vi "Get System Name.vi"() -> (3 "System Name":string)   [LabVIEW 2016]
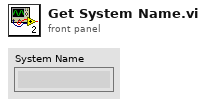
[diagram p1: front panel]
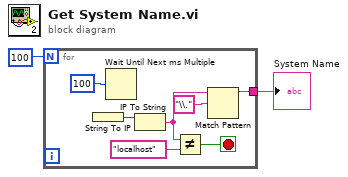
[diagram p0: block diagram]
diagram:
  n1 = for {
    N: 100 -> [_]
    tunnel: [w8] -> w2
    stop <- w5 stop-if-true
    n2 = String To IP() -> (0:w7:u32)  [unwired: 1 in]
    n3 = Wait Until Next ms Multiple(millisecond multiple=u32 100) -> ()  [unwired: 1 out]
    n4 = IP To String(2:w7) -> (0:w4:string)  [unwired: 1 in]
    n5 = Not Equal?(x=w4, y="localhost") -> (x != y?=w5:bool)
    n6 = Match Pattern(string=w4, regular expression="\\.") -> (before substring=w8:string)  [unwired: 1 in, 3 out]
  }
  "System Name" <- w2
